vi "Sample_Data_Subset.vi"(11 "Particle Measurements (Pixels)":dbl[][](array[numeric]) format="%.2f") -> (3 "Sample Data":dbl[](array[numeric]))   [LabVIEW 2022 SP3]
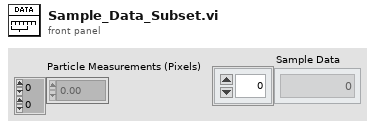
[diagram p1: front panel]
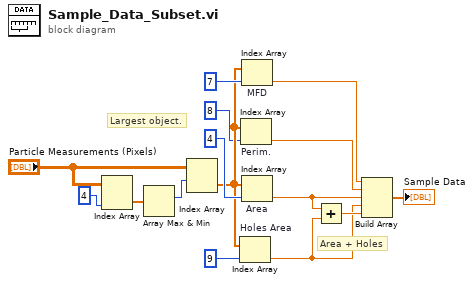
[diagram p0: block diagram]
diagram:
  # "Area + Holes"
  # "Largest object."
  n1 = Index Array(array="Particle Measurements (Pixels)", index (col)=4 ("index (row)")) -> (element=w13:dbl[])  [unwired: 1 in]
  n2 = Array Max & Min(array=w13) -> (max index (indices)=w14:i32)  [unwired: 3 out]
  n3 = Index Array(array="Particle Measurements (Pixels)", index (row)=w14) -> (element=w5:dbl[])  [unwired: 1 in]
  n4 = Index Array "Holes Area"(array=w5, index=9) -> (element=w1:dbl)
  n5 = Index Array "Perim."(array=w5, index=8) -> (element=w3:dbl)
  n6 = Index Array "MFD"(array=w5, index=7) -> (element=w8:dbl)
  n7 = Index Array "Area"(array=w5, index=4) -> (element=w2:dbl)
  n8 = Add(x=w2, y=w1) -> (x+y=w7:dbl)
  n9 = Build Array(w8, w3, w2, w1, w7) -> (→"Sample Data":dbl[])
